vi "FL_Update_Histogram_data.vi"(0 "Histogram count in":u32[](array[numeric]), 1 "Reset? (F)":bool, 2 "Current value":dbl format="%#_13g", 3 "Bins array":dbl[](array[numeric])) -> (5 "Histogram count out":u32[](array[numeric]))   [LabVIEW 2018, in "Tracker.lvlib"]
uses:
  Tracker.lvlib
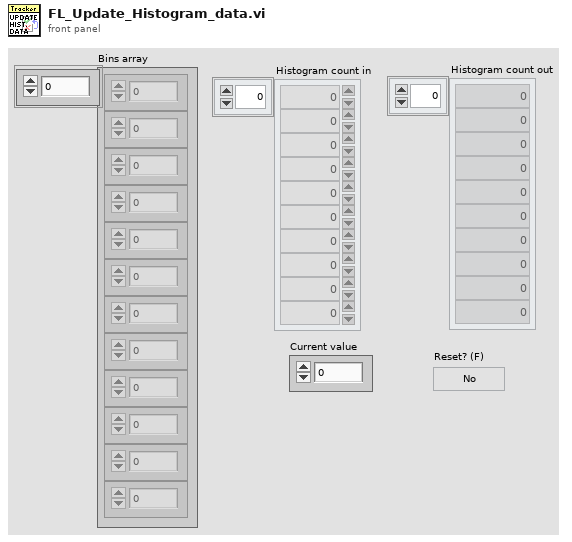
[diagram p1: front panel]
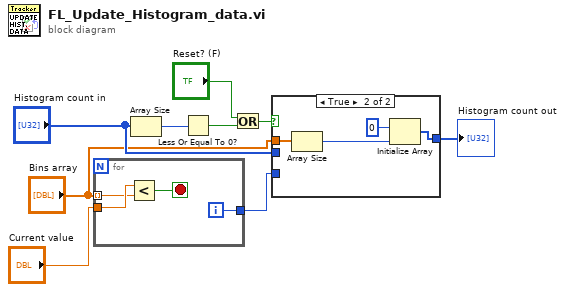
[diagram p0: block diagram]
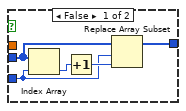
[diagram p2: hidden frame]
diagram:
  n1 = for {
    tunnel: "Bins array" -> [w12] mode=indexing
    tunnel: "Current value" -> [w13]
    tunnel: [w10] -> w2
    i -> [w10]
    stop <- w11 stop-if-true
    n2 = Less?(x=w13, y=w12) -> (x < y?=w11:bool)
  }
  n3 = Array Size(array="Histogram count in") -> (size(s)=w6:i32)
  n4 = Less Or Equal To 0?(x=w6) -> (x <= 0?=w4:bool)
  n5 = Or(x="Reset? (F)", y=w4) -> (x .or. y?=w5:bool)
  n6 = case shown="True" w5 {
    tunnel: [w18 w22] -> w9
    tunnel: w2 -> [w16 _]
    tunnel: "Histogram count in" -> [w15 _]
    tunnel: "Bins array" -> [_ w19]
    frame False {
      n7 = Index Array(array=w15, index=w16) -> (element=w14:u32)
      n8 = Increment(x=w14) -> (x+1=w17:u32)
      n9 = Replace Array Subset(array=w15, new element=w17, index=w16) -> (w18:u32[])
    }
    frame True {
      n10 = Array Size(array=w19) -> (size(s)=w21:i32)
      n11 = Initialize Array(u32 0, w21) -> (w22:u32[])
    }
  }
  "Histogram count out" <- w9
